vi "PGM APP.vi"() -> (2 "standard error":string, 3 "standard output":string)   [LabVIEW 2018]
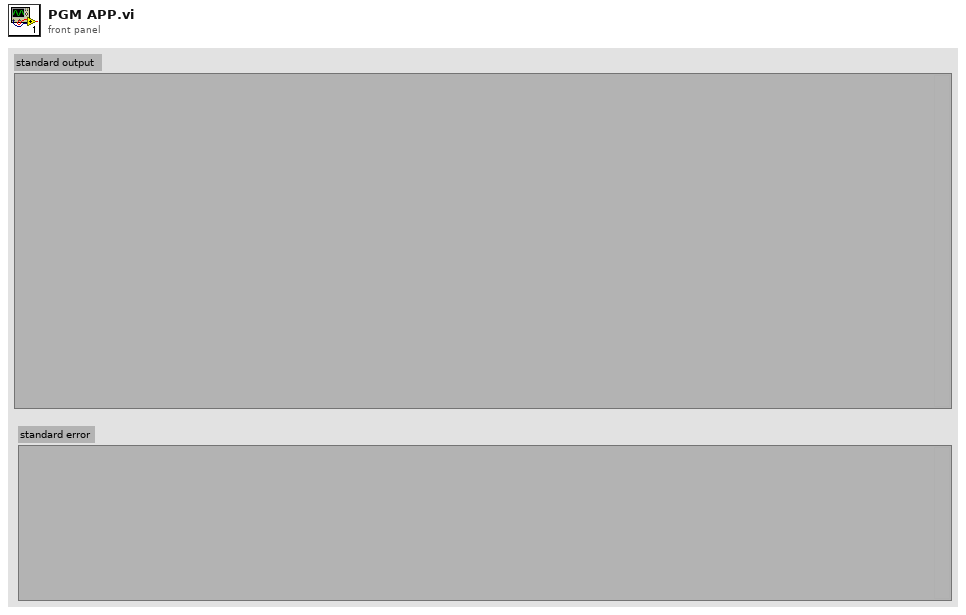
[diagram p1: front panel]
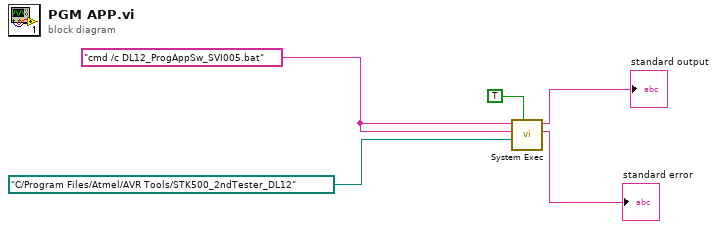
[diagram p0: block diagram]
diagram:
  w2 = "cmd /c DL12_ProgAppSw_SVI005.bat" ("command line")
  n1 = call <vilib>:"System Exec.vi"("wait until completion? (T)"=TRUE, "working directory"=path "C:/Program Files/Atmel/AVR Tools/STK500_2ndTester_DL12", "standard input"=w2, "command line"=w2) -> ("standard error"=→"standard error":string, "standard output"=→"standard output":string)  [unwired: 4 in, 2 out]
